vi "App_User Setting.vi"() -> ()   [LabVIEW 2015, in "Application 2.lvlib"]
uses:
  Application 2.lvlib
panel:
  in  "Remove User":bool caption="Blank"
  out "Login Time":timestamp format="%<%x %.0X>T"
  out "Phone Number":string
  out "Email":string
  out "User Name":string
  out "User Picture":T1(plugin-control)
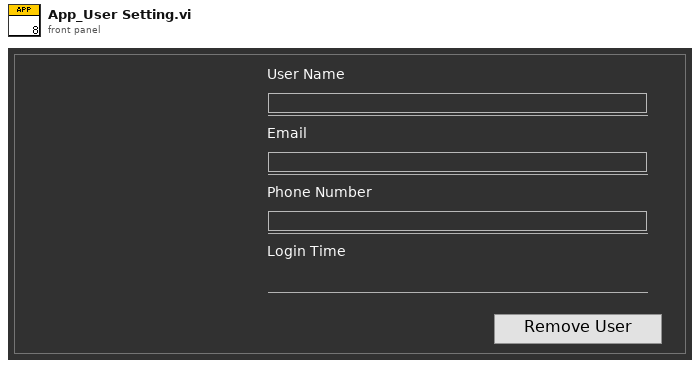
[diagram p1: front panel]
types:
  T1 = typedef "IMAQ Image.ctl" = refnum<image>
  T2 = typedef "Image Type" = u32
  T3 = typedef "Application 2.lvlib/App_Main Data.ctl" = cluster{"VI Refnum":refnum<vi>, "Subpanel":refnum<vi>, "Connection ID":refnum<k5>, "Meta data":T4[], "Main Queue":T6, "User Data":T7}
  T4 = typedef "stm_MetaElement.ctl" = cluster{"Name":T5}
  T5 = typedef "stm_MetaDataElement.ctl" = string
  T6 = typedef "Application 2.lvlib/App_Main Queue.ctl" = cluster{"Main Loop Queue":refnum<queue>}
  T7 = typedef "User Data.ctl" = cluster{"Name":string, "Email":string, "Phone Number":string, "User Picture":u32[][], "Last Login Time":timestamp}
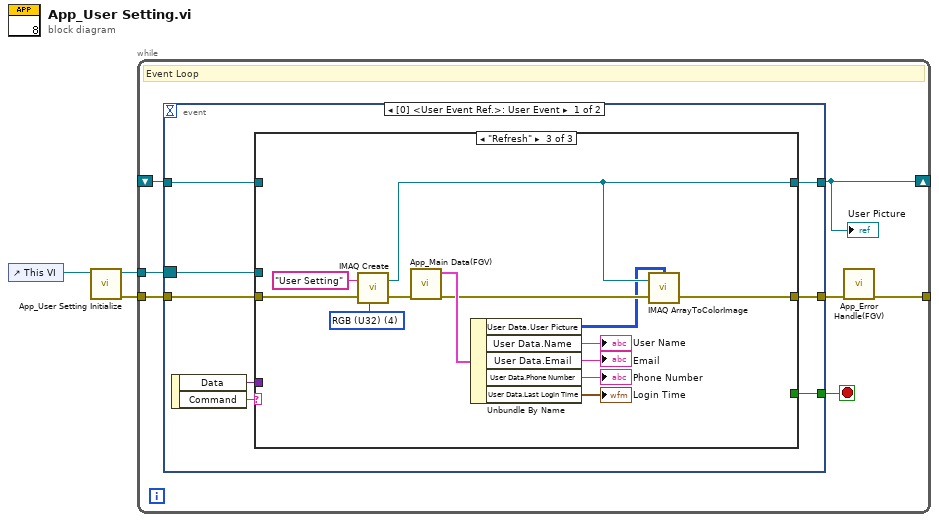
[diagram p0: block diagram]
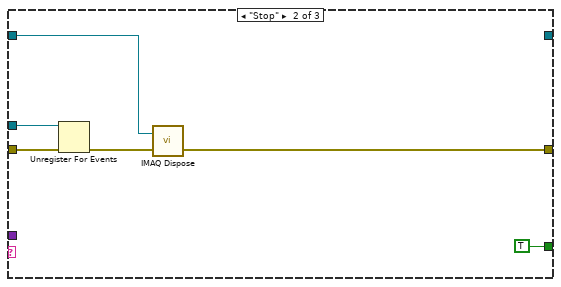
[diagram p3: hidden frame]
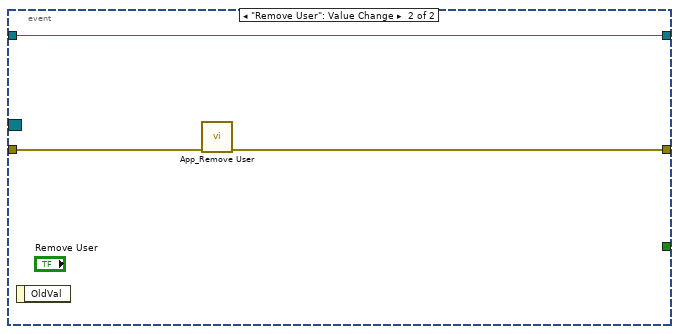
[diagram p4: hidden frame]
diagram:
  n1 = control-ref of="This VI"() -> (w3:refnum<vi>)
  n2 = call "App_User Setting Initialize.vi"("VI Reference"=w3) -> ("error out"=w2:errorcluster, "Event Registration Refnum"=w1:refnum<event-registration>)  [unwired: 9 in]
  n3 = while {
    tunnel: w2 -> [w10]
    tunnel: w1 -> [w9]
    tunnel: [w7] -> _
    shift-right: [w4] -> _
    shift-left: _ -> [w5]
    stop <- w6 stop-if-true
    # "Event Loop"
    n4 = event shown="[0] <User Event Ref.>: User Event" {
      selector: w9 -> [w15 _]
      dyn-events: _ -> [_ _]
      timeout: _ -> [_ _]
      tunnel: w10 -> [w16 w41]
      tunnel: [w14 w40] -> w8
      tunnel: [w13 _] -> w6
      tunnel: [w12 w42] -> w4
      tunnel: w5 -> [w11 w42]
      event User Event {
        n5 = event-data() -> ("Data"=w17:variant, "Command"=w18:string)  [unwired: 1 in]
        n6 = case shown="\"Refresh\"" w18 {
          tunnel: w17 -> [_ _ _]
          tunnel: w16 -> [w20 w26 w39]
          tunnel: w15 -> [_ w25 _]
          tunnel: [w20 w21 w31] -> w14
          tunnel: [_ TRUE _] -> w13
          tunnel: [w19 _ w33] -> w12
          tunnel: w11 -> [w19 w22 _]
          frame Default {
          }
          frame "Stop" {
            n7 = Unregister For Events(event registration refnum=w25, error in=w26) -> (error out=w23:errorcluster)
            n8 = call "IMAQ Dispose"("Image"=w22, "error in (no error)"=w23) -> ("error out"=w21:errorcluster)  [unwired: 4 in]
          }
          frame "Refresh" {
            w37 = T2 4 items=["Grayscale (U8)", "Grayscale (I16)", "Grayscale (SGL)", "Complex (CSG)", "RGB (U32)", "HSL (U32)", "RGB (U64)", "Grayscale (U16)"] ("Image Type")
            n9 = call "IMAQ Create"("Image Name"="User Setting", "Image Type"=w37, "error in (no error)"=w39) -> ("New Image"=w33:T1, "error out"=w36:errorcluster)  [unwired: 2 in]
            n10 = call "App_Main Data(FGV).vi"("error in"=w36) -> ("error out"=w34:errorcluster, "Main Data Out"=w35:T3)  [unwired: 9 in]
            n11 = Unbundle By Name(w35) -> ("User Data.User Picture"=w32:u32[][], "User Data.Name"=→"User Name":string, "User Data.Email"=→"Email":string, "User Data.Phone Number"=→"Phone Number":string, "User Data.Last Login Time"=→"Login Time":timestamp)
            n12 = call "IMAQ ArrayToColorImage"("Image Pixels (U32)"=w32, "Image"=w33, "error in (no error)"=w34) -> ("error out"=w31:errorcluster)  [unwired: 2 in, 1 out]
          }
        }
      }
      event "Remove User": Value Change {
        n13 = event-data() -> ()  [unwired: 1 in, 1 out]
        n14 = call "App_Remove User.vi"("error in"=w41) -> ("error out"=w40:errorcluster)  [unwired: 10 in]
      }
    }
    "User Picture" <- w4
    n15 = call "App_Error Handle(FGV).vi"("error in"=w8) -> ("error out"=w7:errorcluster)  [unwired: 9 in, 1 out]
  }
